vi "grow_pops.vi"(4 "rho- condition":dbl[](array[numeric]), 5 "Decay rate":dbl, 6 "rho0 condition":dbl[](array[numeric]), 7 "Microwave power":dbl, 8 "rho+ condition":dbl[](array[numeric]), 9 "rho- array":dbl[](array[numeric]), 10 "rho0 array":dbl[](array[numeric]), 11 "rho+ array":dbl[](array[numeric])) -> (1 "rho- array out":dbl[](array[numeric]), 2 "rho0 array out":dbl[](array[numeric]), 3 "rho+ array out":dbl[](array[numeric]))   [LabVIEW 2018]
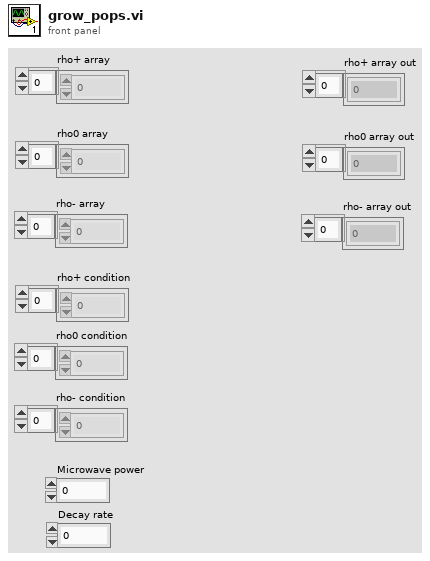
[diagram p1: front panel]
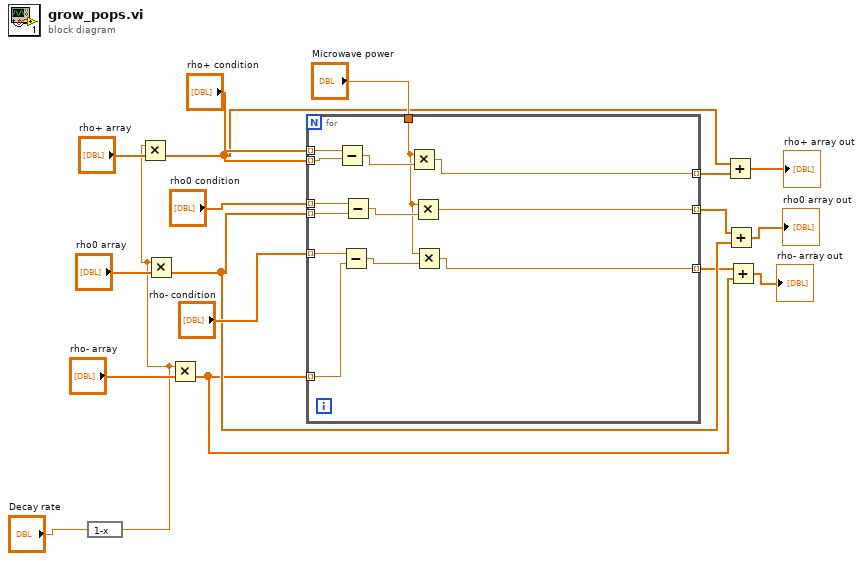
[diagram p0: block diagram]
diagram:
  n1 = expression code="1-x"("Decay rate") -> (w11:dbl)
  n2 = Multiply(x=w11, y="rho+ array") -> (x*y=w9:dbl[])
  n3 = Multiply(x=w11, y="rho0 array") -> (x*y=w6:dbl[])
  n4 = Multiply(x=w11, y="rho- array") -> (x*y=w5:dbl[])
  n5 = for {
    tunnel: "rho+ condition" -> [w31] mode=indexing
    tunnel: "rho0 condition" -> [w30] mode=indexing
    tunnel: w6 -> [w29] mode=indexing
    tunnel: w9 -> [w28] mode=indexing
    tunnel: "rho- condition" -> [w27] mode=indexing
    tunnel: w5 -> [w26] mode=indexing
    tunnel: "Microwave power" -> [w22]
    tunnel: [w21] -> w8 mode=indexing
    tunnel: [w20] -> w7 mode=indexing
    tunnel: [w19] -> w4 mode=indexing
    n6 = Subtract(x=w31, y=w28) -> (x-y=w23:dbl)
    n7 = Subtract(x=w27, y=w26) -> (x-y=w25:dbl)
    n8 = Subtract(x=w30, y=w29) -> (x-y=w24:dbl)
    n9 = Multiply(x=w22, y=w23) -> (x*y=w21:dbl)
    n10 = Multiply(x=w22, y=w24) -> (x*y=w20:dbl)
    n11 = Multiply(x=w22, y=w25) -> (x*y=w19:dbl)
  }
  n12 = Add(x=w9, y=w8) -> (x+y=→"rho+ array out":dbl[])
  n13 = Add(x=w7, y=w6) -> (x+y=→"rho0 array out":dbl[])
  n14 = Add(x=w4, y=w5) -> (x+y=→"rho- array out":dbl[])
